vi "aplication 1.vi"() -> ()   [LabVIEW 2019]
panel:
  out "temps mis":u32
  out "XY Graph":cluster{dbl[], dbl[]}(graph)
  out "Waveform Graph":dbl[](graph)
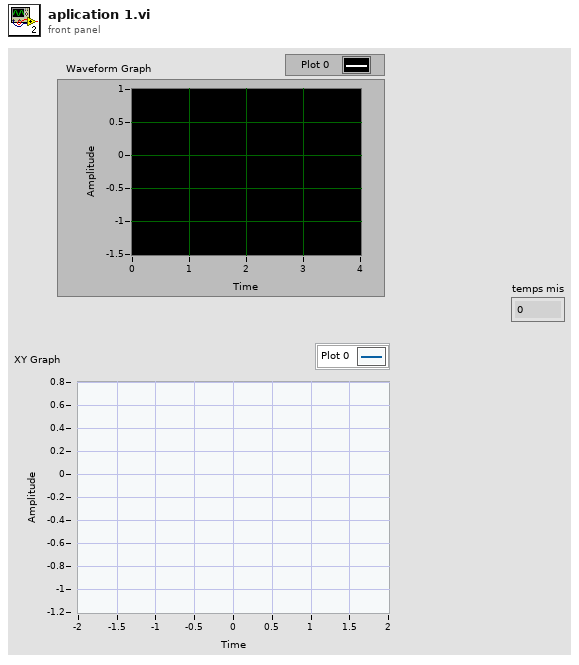
[diagram p1: front panel]
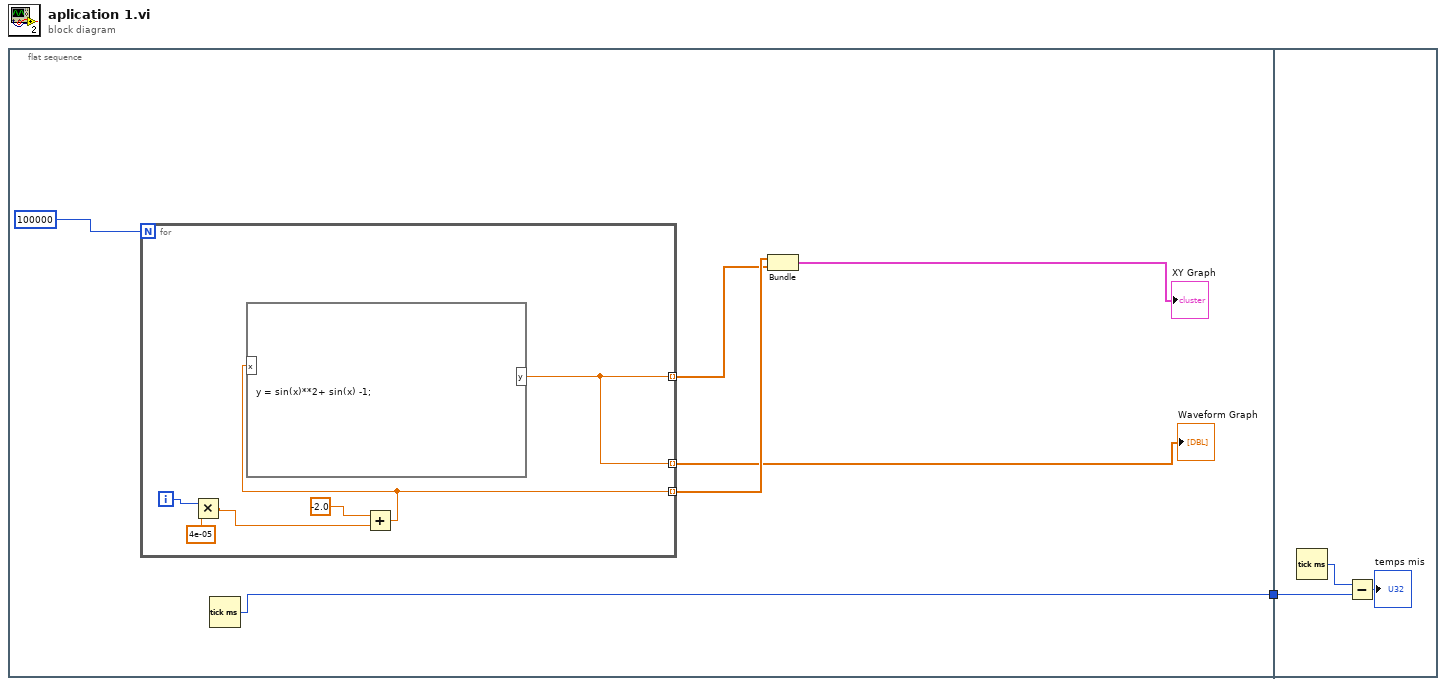
[diagram p0: block diagram]
diagram:
  n1 = flat-sequence {
    tunnel: [w2] -> w1
    tunnel: w1 -> [w15]
    frame #0 {
      n2 = for {
        N: 100000 -> [_]
        tunnel: [w12] -> w6 mode=indexing
        tunnel: [w11] -> w5 mode=indexing
        tunnel: [w11] -> w4 mode=indexing
        i -> [w10]
        n3 = Multiply(x=w10, y=4e-05) -> (x*y=w8:dbl)
        n4 = Add(x=-2.0, y=w8) -> (x+y=w12:dbl)
        n5 = formula code="y = sin(x)**2+ sin(x) -1;"("x"=w12) -> ("y"=w11:dbl)
      }
      "Waveform Graph" <- w4
      n6 = Tick Count (ms)() -> (millisecond timer value=w2:u32)
      n7 = Bundle(w6, w5) -> (→"XY Graph":cluster{dbl[], dbl[]})  [unwired: 1 in]
    }
    frame #1 {
      n8 = Tick Count (ms)() -> (millisecond timer value=w16:u32)
      n9 = Subtract(x=w16, y=w15) -> (x-y=→"temps mis":u32)
    }
  }
